vi "test_12.vi"() -> ()   [LabVIEW 2017]
uses:
  <vilib>/measure/maspectr.llb/FFT Power Spectrum and PSD for 1 Chan.vi
  <vilib>/measure/NI_MABase.lvlib
  <vilib>/measure/NI_MAPro.lvlib
  <vilib>/Analysis/NI_AALBase.lvlib
panel:
  out "TX Spectrum 2":cluster{"f0":dbl, "df":dbl, "magnitude":dbl[]}(graph)
  out "TX Signal 6":waveform(dbl)(graph)
  out "phase out 2":dbl caption="위상 출력" format="%0.2e"
  out "phase out":dbl caption="위상 출력" format="%0.2e"
  out "TX Signal 5":waveform(dbl)(graph)
  out "TX Spectrum":cluster{"f0":dbl, "df":dbl, "magnitude":dbl[]}(graph)
  out "TX Signal 4":waveform(dbl)(graph)
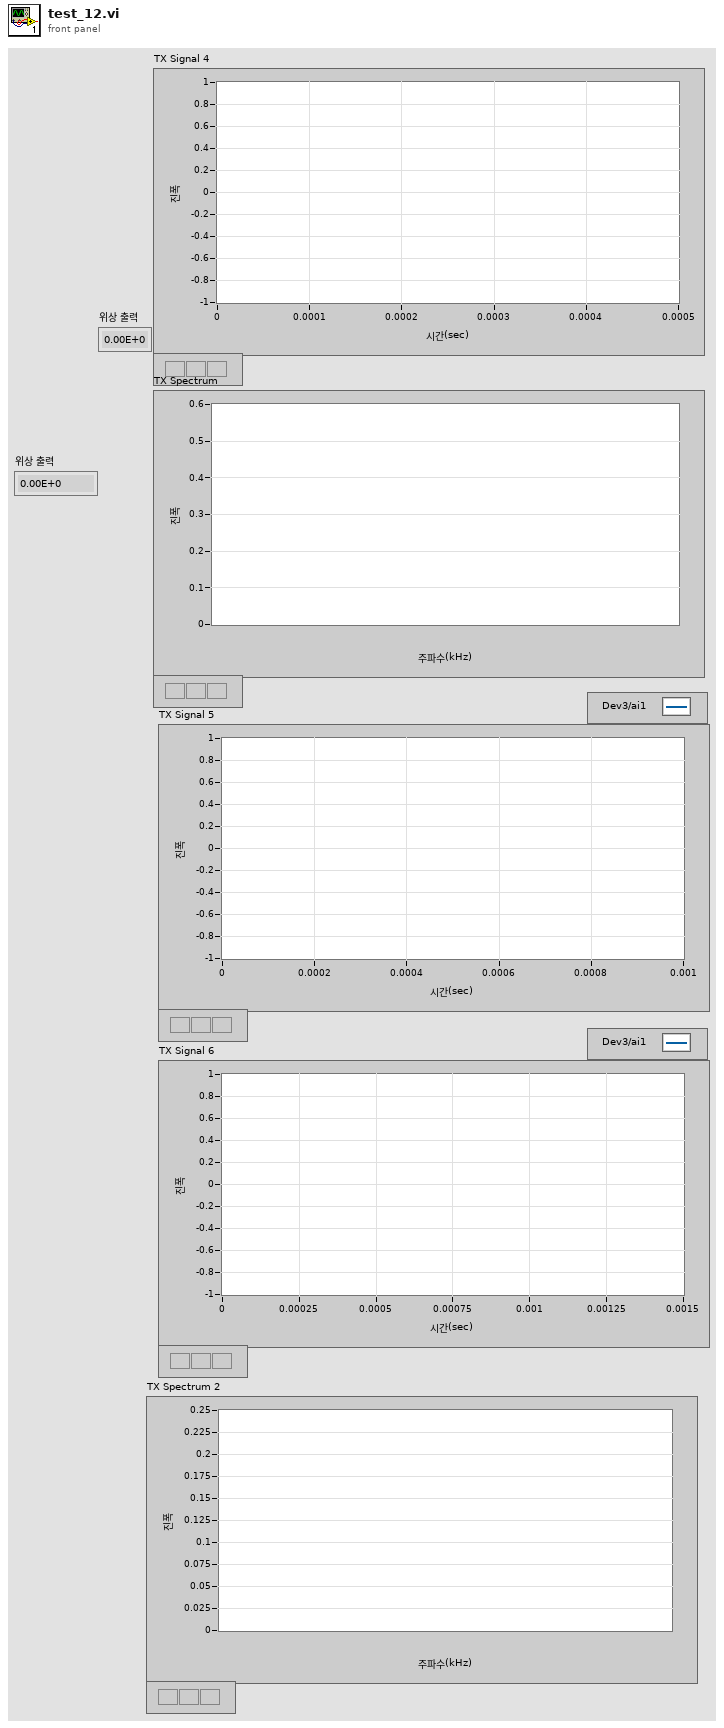
[diagram p1: front panel]
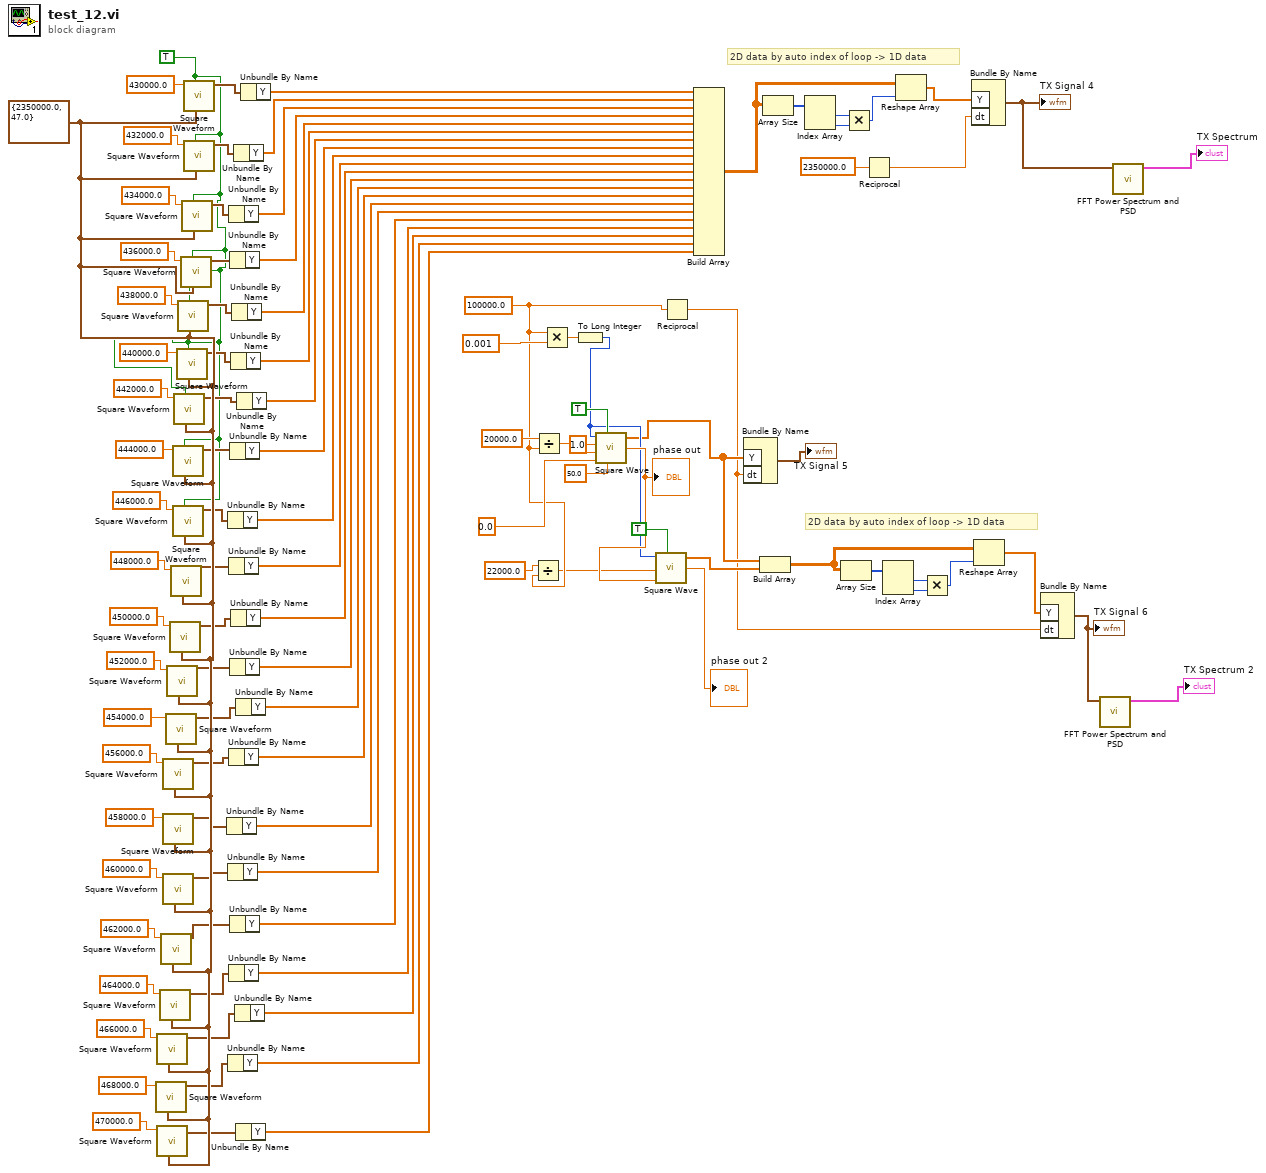
[diagram p0: block diagram]
diagram:
  w15 = 100000.0 ("x")
  w29 = TRUE ("reset signal")
  w78 = cluster{"Fs":dbl, "#s":dbl} {"Fs"=2350000.0, "#s"=47.0} ("sampling info")
  # "2D data by auto index of loop -> 1D data"
  # "2D data by auto index of loop -> 1D data"
  n1 = call <vilib>:"Square Waveform.vi"("sampling info"=w78, "frequency"=468000.0) -> ("signal out"=w58:waveform(dbl))  [unwired: 8 in, 1 out]
  n2 = call <vilib>:"Square Waveform.vi"("sampling info"=w78, "frequency"=466000.0) -> ("signal out"=w59:waveform(dbl))  [unwired: 8 in, 1 out]
  n3 = call <vilib>:"Square Waveform.vi"("sampling info"=w78, "frequency"=470000.0) -> ("signal out"=w57:waveform(dbl))  [unwired: 8 in, 1 out]
  n4 = call <vilib>:"Square Waveform.vi"("sampling info"=w78, "frequency"=464000.0) -> ("signal out"=w60:waveform(dbl))  [unwired: 8 in, 1 out]
  n5 = call <vilib>:"Square Waveform.vi"("sampling info"=w78, "frequency"=462000.0) -> ("signal out"=w61:waveform(dbl))  [unwired: 8 in, 1 out]
  n6 = call <vilib>:"Square Waveform.vi"("sampling info"=w78, "frequency"=456000.0) -> ("signal out"=w64:waveform(dbl))  [unwired: 8 in, 1 out]
  n7 = call <vilib>:"Square Waveform.vi"("sampling info"=w78, "frequency"=458000.0) -> ("signal out"=w63:waveform(dbl))  [unwired: 8 in, 1 out]
  n8 = call <vilib>:"Square Waveform.vi"("sampling info"=w78, "frequency"=460000.0) -> ("signal out"=w62:waveform(dbl))  [unwired: 8 in, 1 out]
  n9 = call <vilib>:"Square Waveform.vi"("sampling info"=w78, "frequency"=454000.0) -> ("signal out"=w65:waveform(dbl))  [unwired: 8 in, 1 out]
  n10 = call <vilib>:"Square Waveform.vi"("sampling info"=w78, "frequency"=452000.0) -> ("signal out"=w66:waveform(dbl))  [unwired: 8 in, 1 out]
  n11 = call <vilib>:"Square Waveform.vi"("sampling info"=w78, "frequency"=450000.0) -> ("signal out"=w67:waveform(dbl))  [unwired: 8 in, 1 out]
  n12 = call <vilib>:"Square Waveform.vi"("sampling info"=w78, "frequency"=448000.0) -> ("signal out"=w68:waveform(dbl))  [unwired: 8 in, 1 out]
  n13 = call <vilib>:"Square Waveform.vi"("sampling info"=w78, "reset signal"=w29, "frequency"=444000.0) -> ("signal out"=w70:waveform(dbl))  [unwired: 7 in, 1 out]
  n14 = call <vilib>:"Square Waveform.vi"("sampling info"=w78, "reset signal"=w29, "frequency"=446000.0) -> ("signal out"=w69:waveform(dbl))  [unwired: 7 in, 1 out]
  n15 = call <vilib>:"Square Waveform.vi"("sampling info"=w78, "reset signal"=w29, "frequency"=442000.0) -> ("signal out"=w71:waveform(dbl))  [unwired: 7 in, 1 out]
  n16 = call <vilib>:"Square Waveform.vi"("sampling info"=w78, "reset signal"=w29, "frequency"=440000.0) -> ("signal out"=w72:waveform(dbl))  [unwired: 7 in, 1 out]
  n17 = call <vilib>:"Square Waveform.vi"("sampling info"=w78, "reset signal"=w29, "frequency"=438000.0) -> ("signal out"=w73:waveform(dbl))  [unwired: 7 in, 1 out]
  n18 = call <vilib>:"Square Waveform.vi"("sampling info"=w78, "reset signal"=w29, "frequency"=436000.0) -> ("signal out"=w74:waveform(dbl))  [unwired: 7 in, 1 out]
  n19 = call <vilib>:"Square Waveform.vi"("sampling info"=w78, "reset signal"=w29, "frequency"=434000.0) -> ("signal out"=w75:waveform(dbl))  [unwired: 7 in, 1 out]
  n20 = call <vilib>:"Square Waveform.vi"("sampling info"=w78, "reset signal"=w29, "frequency"=430000.0) -> ("signal out"=w77:waveform(dbl))  [unwired: 7 in, 1 out]
  n21 = call <vilib>:"Square Waveform.vi"("sampling info"=w78, "reset signal"=w29, "frequency"=432000.0) -> ("signal out"=w76:waveform(dbl))  [unwired: 7 in, 1 out]
  n22 = Unbundle By Name(w63) -> ("Y"=w42:dbl[])
  n23 = Unbundle By Name(w69) -> ("Y"=w48:dbl[])
  n24 = Unbundle By Name(w62) -> ("Y"=w41:dbl[])
  n25 = Unbundle By Name(w58) -> ("Y"=w37:dbl[])
  n26 = Unbundle By Name(w75) -> ("Y"=w54:dbl[])
  n27 = Unbundle By Name(w68) -> ("Y"=w47:dbl[])
  n28 = Unbundle By Name(w64) -> ("Y"=w43:dbl[])
  n29 = Unbundle By Name(w60) -> ("Y"=w39:dbl[])
  n30 = Unbundle By Name(w74) -> ("Y"=w53:dbl[])
  n31 = Unbundle By Name(w70) -> ("Y"=w49:dbl[])
  n32 = Unbundle By Name(w66) -> ("Y"=w45:dbl[])
  n33 = Unbundle By Name(w61) -> ("Y"=w40:dbl[])
  n34 = Unbundle By Name(w72) -> ("Y"=w51:dbl[])
  n35 = Unbundle By Name(w67) -> ("Y"=w46:dbl[])
  n36 = Unbundle By Name(w73) -> ("Y"=w52:dbl[])
  n37 = Unbundle By Name(w76) -> ("Y"=w55:dbl[])
  n38 = Unbundle By Name(w59) -> ("Y"=w38:dbl[])
  n39 = Unbundle By Name(w65) -> ("Y"=w44:dbl[])
  n40 = Unbundle By Name(w57) -> ("Y"=w36:dbl[])
  n41 = Unbundle By Name(w71) -> ("Y"=w50:dbl[])
  n42 = Unbundle By Name(w77) -> ("Y"=w56:dbl[])
  n43 = Divide(x=22000.0, y=w15) -> (x/y=w14:dbl)
  n44 = Divide(x=20000.0, y=w15) -> (x/y=w20:dbl)
  n45 = Multiply(x=w15, y=0.001) -> (x*y=w26:dbl)
  n46 = To Long Integer(number=w26) -> (32bit integer=w17:i32)
  n47 = call <vilib>:"Square Wave.vi"("samples"=w17, "reset phase"=TRUE, "amplitude"=1.0, "frequency"=w20, "duty cycle (%)"=50.0, "phase in"=0.0) -> ("square wave"=w12:dbl[], "phase out"=w18:dbl)  [unwired: 1 out]
  "phase out" <- w18
  n48 = call <vilib>:"Square Wave.vi"("samples"=w17, "reset phase"=TRUE, "frequency"=w14, "phase in"=w18) -> ("square wave"=w11:dbl[], "phase out"=→"phase out 2":dbl)  [unwired: 2 in, 1 out]
  n49 = Reciprocal(x=w15) -> (1/x=w4:dbl)
  n50 = Build Array(w56, w55, w54, w53, w52, w51, w50, w49, w48, w47, w46, w45, w44, w43, w42, w41, w40, w39, w38, w37, w36) -> (w35:dbl[][])
  n51 = Bundle By Name("Y"=w12, "dt"=w4) -> (→"TX Signal 5":waveform(dbl))  [unwired: 1 in]
  n52 = Build Array(w12, w11) -> (w6:dbl[][])
  n53 = Array Size(array=w35) -> (size(s)=w34:i32[])
  n54 = Index Array(array=w34) -> (element #1=w33:i32, element #2=w32:i32)  [unwired: 2 in]
  n55 = Array Size(array=w6) -> (size(s)=w9:i32[])
  n56 = Multiply(x=w33, y=w32) -> (x*y=w102:i32)
  n57 = Reciprocal(x=2350000.0 ("Fs")) -> (1/x=w28:dbl)
  n58 = Index Array(array=w9) -> (element #1=w8:i32, element #2=w7:i32)  [unwired: 2 in]
  n59 = Reshape Array(w35, w102) -> (w31:dbl[])
  n60 = Multiply(x=w8, y=w7) -> (x*y=w10:i32)
  n61 = Bundle By Name("Y"=w31, "dt"=w28) -> (w101:waveform(dbl))  [unwired: 1 in]
  "TX Signal 4" <- w101
  n62 = Reshape Array(w6, w10) -> (w5:dbl[])
  n63 = Bundle By Name("Y"=w5, "dt"=w4) -> (w1:waveform(dbl))  [unwired: 1 in]
  "TX Signal 6" <- w1
  n64 = call-poly <vilib>:"FFT Power Spectrum and PSD.vi"("time signal"=w1) -> ("Power Spectrum / PSD"=→"TX Spectrum 2":cluster{"f0":dbl, "df":dbl, "magnitude":dbl[]})  [unwired: 7 in, 3 out]
  n65 = call-poly <vilib>:"FFT Power Spectrum and PSD.vi"("time signal"=w101) -> ("Power Spectrum / PSD"=→"TX Spectrum":cluster{"f0":dbl, "df":dbl, "magnitude":dbl[]})  [unwired: 7 in, 3 out]
